vi "YAxisOutputs (1).vi"(8 "error in (no error)":errorcluster, 9 "PWM  Frequency Command (Hz)":dbl, 10 "YActiveDirectionCmd":bool, 11 "Y-Axis Direction Request":bool) -> (0 "error out":errorcluster, 2 "Limited Output":dbl, 3 "Direction Command":bool)   [LabVIEW 2013]
uses:
  <vilib>/myRIO/Instrument Drivers/Onboard IO/PWM/vis/Smart Open.vi
  <vilib>/myRIO/Instrument Drivers/Onboard IO/PWM/vis/Set Duty Cycle and Frequency.vi
  <vilib>/myRIO/Instrument Drivers/Onboard IO/DIO/vis/Smart Open.vi
  <vilib>/myRIO/Instrument Drivers/Onboard IO/DIO/vis/Write.vi
  <vilib>/myRIO/Instrument Drivers/Onboard IO/PWM/vis/Open.vi
  <vilib>/myRIO/Instrument Drivers/Onboard IO/DIO/vis/Open.vi
  <vilib>/myRIO/Common/Instrument Driver Framework/myRIO v1.0/PWM/vis/myRIO v1.1 Open PWM.vi
  <vilib>/myRIO/Common/Instrument Driver Framework/myRIO v1.0/DIO/vis/myRIO v1.1 Open DIO.vi
  <vilib>/myRIO/Common/Instrument Driver Framework/Utilities/vis/Validate Channels.vi
  <vilib>/myRIO/Common/Instrument Driver Framework/myRIO v1.0/PWM/vis/myRIO v1.0 Reserve PWM.vi
  <vilib>/myRIO/Common/Instrument Driver Framework/myRIO v1.0/DIO/vis/myRIO v1.0 Reserve DIO.vi
  <vilib>/myRIO/Common/Instrument Driver Framework/myRIO v1.0/PWM/vis/myRIO v1.0 Build MUX Configuration PWM.vi
  <vilib>/myRIO/Common/Instrument Driver Framework/myRIO v1.0/Resource Manager/vis/myRIO v1.0 Reserve Channel List.vi
  <vilib>/myRIO/Common/Instrument Driver Framework/myRIO v1.0/DIO/vis/myRIO v1.0 Build MUX Configuration DIO.vi
  <vilib>/myRIO/Common/Instrument Driver Framework/myRIO v1.0/Resource Manager/vis/myRIO v1.0 Create Configuration List.vi
  <vilib>/myRIO/Common/Instrument Driver Framework/myRIO v1.0/Resource Manager/vis/myRIO v1.0 Reserve Channel.vi
  <vilib>/myRIO/Common/Instrument Driver Framework/myRIO v1.0/Resource Manager/vis/myRIO v1.0 Unreserve Channel.vi
  <vilib>/myRIO/Common/Instrument Driver Framework/myRIO v1.0/Resource Manager/vis/myRIO v1.0 Build Mutex Name.vi
  <vilib>/addons/control/pid/pid.llb/PID Output Rate Limiter (DBL).vi
  <vilib>/myRIO/Common/Instrument Driver Framework/myRIO v1.0/myRIO v1.1 Open.vi
  <vilib>/Utility/VariantDataType/GetNumericInfo.vi
  <vilib>/Utility/error.llb/Error Cluster From Error Code.vi
  <vilib>/myRIO/Common/Instrument Driver Framework/Utilities/vis/IO Manager.vi
  <vilib>/myRIO/Common/Instrument Driver Framework/Utilities/vis/Configuration Manager.vi
  <vilib>/myRIO/Common/Instrument Driver Framework/myRIO v1.0/Resource Manager/vis/myRIO v1.0 Configure IO.vi
  <vilib>/myRIO/Common/Instrument Driver Framework/myRIO v1.0/myRIO v1.0 Close.vi
  <vilib>/myRIO/Common/Instrument Driver Framework/myRIO v1.0/DIO/vis/myRIO v1.0 Write DIO.vi
  <vilib>/myRIO/Common/Instrument Driver Framework/myRIO v1.0/PWM/vis/myRIO v1.0 Write PWM.vi
  <vilib>/addons/control/pid/NI_PID_pid.lvlib
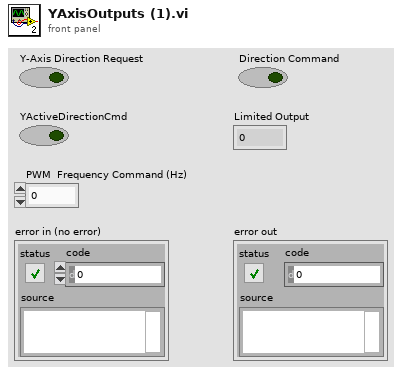
[diagram p1: front panel]
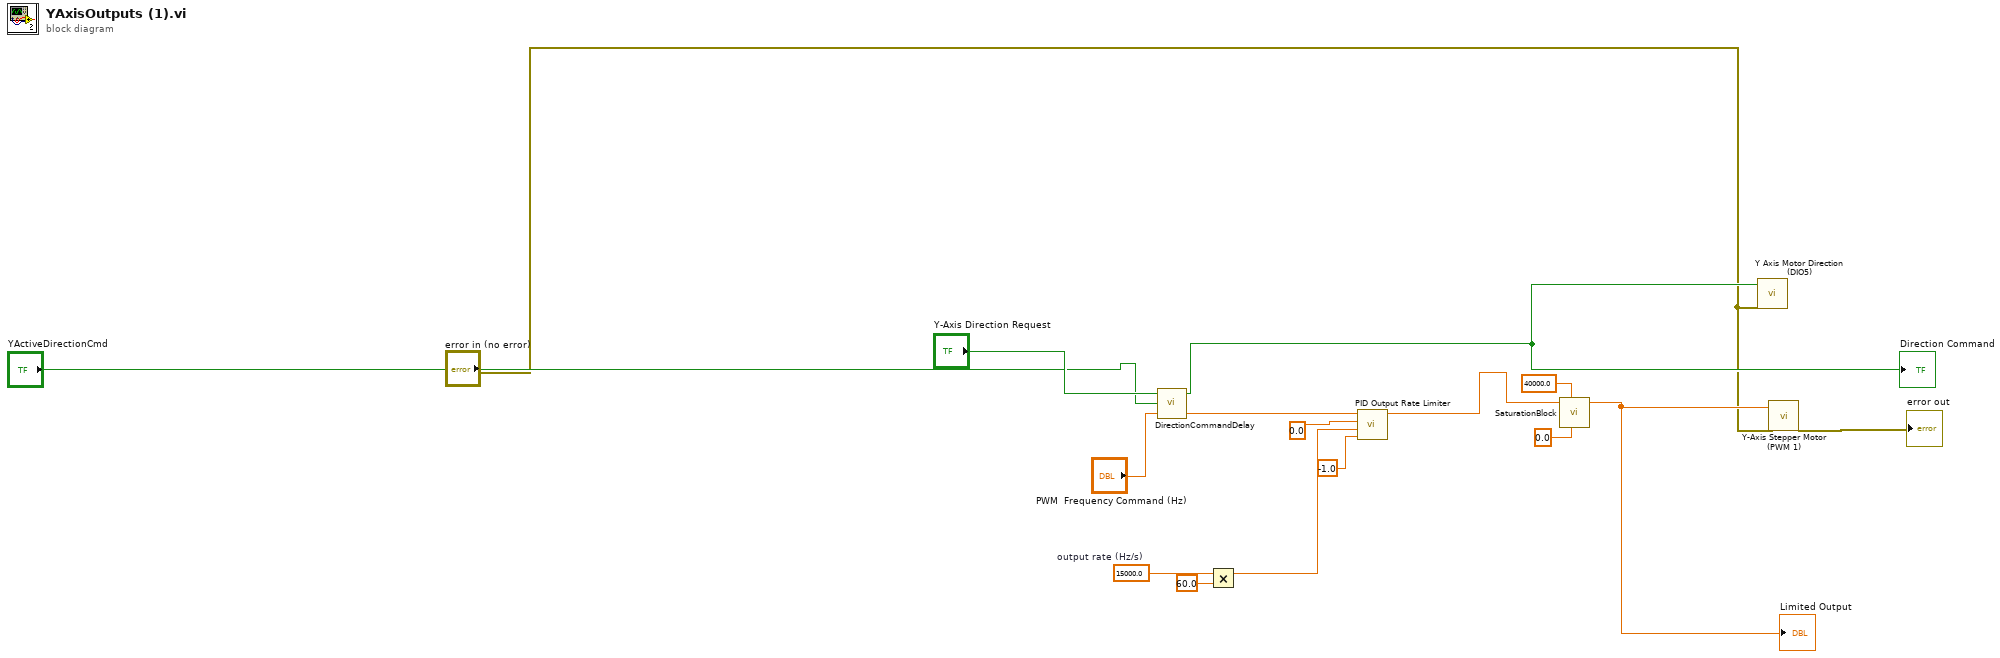
[diagram p0: block diagram]
diagram:
  w5 = 15000.0  # output rate (Hz/s)
  n1 = call "DirectionCommandDelay.vi"("Motor PWM Request"="PWM  Frequency Command (Hz)", "Current Direction"="YActiveDirectionCmd", "Direction Request"="Y-Axis Direction Request") -> ("Motor PWM Command"=w7:dbl, "Direction Command"=w16:bool)  [unwired: 1 out]
  "Direction Command" <- w16
  n2 = Multiply(x=w5, y=60.0) -> (x*y=w2:dbl)
  n3 = call-poly <vilib>:"PID Output Rate Limiter.vi"("dt (s)"=-1.0, "output rate (EGU/min)"=w2, "initial output"=0.0, "input (controller output)"=w7) -> ("output"=w3:dbl)  [unwired: 4 in, 1 out]
  n4 = call "SaturationBlock.vi"("Lower Limit"=0.0, "Upper Limit"=40000.0, "Input"=w3) -> ("Limited Output"=w15:dbl)  [unwired: 8 in]
  "Limited Output" <- w15
  n5 = call "Y Axis Motor Direction (DIO5)"("Y-Axis Direction (A/DIO5 (Pin 21))"=w16, "error in (no error)"="error in (no error)") -> ()  [unwired: 25 in, 1 out]
  n6 = call "Y-Axis Stepper Motor (PWM 1)"("Frequency (Hz)"=w15, "error in (no error)"="error in (no error)") -> ("error out"=→"error out":errorcluster)  [unwired: 25 in]
